vi "Set Solenoid.vi"(8 "error in (no error)":errorcluster, 10 "Value":T1, 11 "Solenoids":T2) -> (0 "error out":errorcluster)   [LabVIEW 2015]
uses:
  Solenoids.ctl
  <vilib>/Rock Robotics/WPI/Solenoid/WPI_SolenoidValue.ctl
  Solenoid Global.vi
  <vilib>/Rock Robotics/WPI/Solenoid/WPI_SolenoidSetEnum.vi
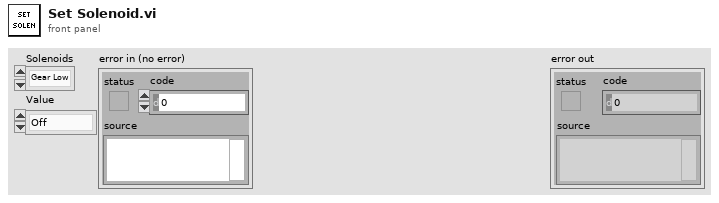
[diagram p1: front panel]
types:
  T1 = typedef "WPI_SolenoidValue.ctl" = enum16{"Off", "On", "Forward", "Reverse"}
  T2 = typedef "Solenoids.ctl" = enum16{"Gear Low", "Gear High", "Shoot Ball", "Hold Ball", "PTO Active", "PTO De-Active"}
  T3 = typedef "WPI_SolenoidDevRef.ctl" = cluster{"DevStatus":errorcluster, "Pneumatics Control Module":u8, "Forward Solenoid Channel":T4, "Reverse Solenoid Channel":T4}
  T4 = typedef "WPI_SolenoidChannel.ctl" = enum8{"Solenoid 0", "Solenoid 1", "Solenoid 2", "Solenoid 3", "Solenoid 4", "Solenoid 5", "Solenoid 6", "Solenoid 7", "Invalid"}
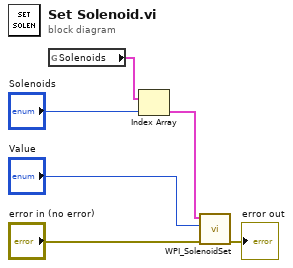
[diagram p0: block diagram]
diagram:
  n1 = global read "Solenoid Global.vi" "Solenoids"() -> (w6:T3[])
  n2 = Index Array(array=w6, index="Solenoids") -> (element=w4:T3)
  n3 = call-poly <vilib>:"WPI_SolenoidSet.vi"("error in (no error)"="error in (no error)", "Value"="Value", "SolenoidDevRef"=w4) -> ("error out"=→"error out":errorcluster)  [unwired: 7 in, 1 out]
